vi "Dialog box.vi"(0 "Missing Str":string) -> (7 "Response":T1(ring))   [LabVIEW 2016]
panel:
  in  "Cancel Button":bool
  in  "new only":bool
  in  "All+ remove old":bool
  in  "All+keep old":bool
  out "Missing Str":string
  # "Some valve ratios have already been calibrated.\nThe following are still missing:"
  # "How would you like to proceed?"
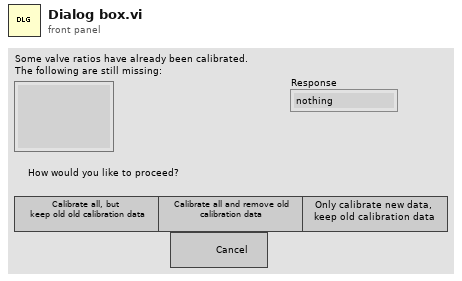
[diagram p1: front panel]
types:
  T1 = enum16{"nothing", "All + Keep Old", "All + Remove Old", "Nothing", "New Only", "Nothin3", "Nothing4", "Nothing5", "Cancel"}
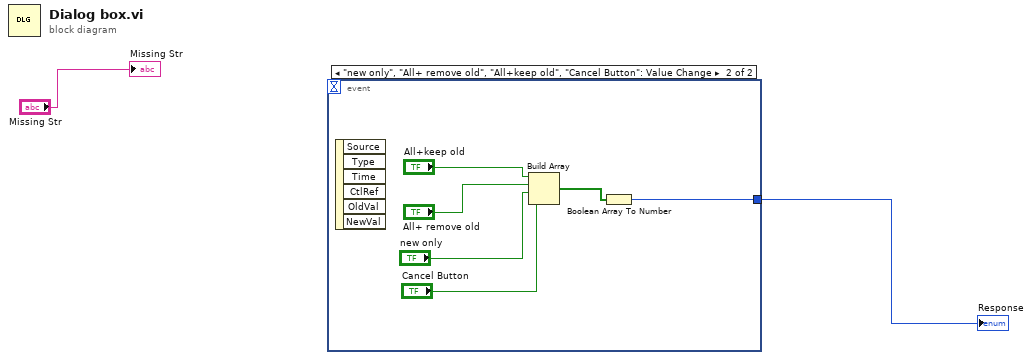
[diagram p0: block diagram]
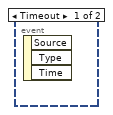
[diagram p2: hidden frame]
diagram:
  n1 = event shown="[1] \"new only\", \"All+ remove old\", \"All+keep old\", \"Cancel Button\": Value Change" {
    selector: _ -> [_ _]
    dyn-events: _ -> [_ _]
    timeout: _ -> [_ _]
    tunnel: [_ w3] -> w1
    event Timeout {
      n2 = event-data() -> ()  [unwired: 1 in, 3 out]
    }
    event "new only", "All+ remove old", "All+keep old", "Cancel Button": Value Change {
      n3 = event-data() -> ()  [unwired: 1 in, 6 out]
      n4 = Build Array("All+keep old", "All+ remove old", "new only", "Cancel Button") -> (w5:bool[])
      n5 = Boolean Array To Number(Boolean array=w5) -> (number=w3:u32)
    }
  }
  "Response" <- w1
  "Missing Str" <- "Missing Str"
